vi "M02 Toy Factory.vi"(9 "Angle in":dbl format="%#_13g", 11 "EV3 in":T1) -> (3 "EV3 out":T1)   [LabVIEW 2016]
uses:
  <vilib>/NXT/Subs/LVHSConnector.ctl
  <vilib>/NXT/LegoClasses/BrickReference/BrickReference.lvclass
  <vilib>/NXT/Dual Mode Library/Waits/Wait_Num.vi
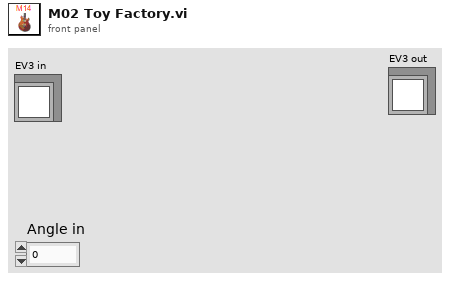
[diagram p1: front panel]
types:
  T1 = typedef "LVHSConnector.ctl" = refnum<class "BrickReference.lvclass">
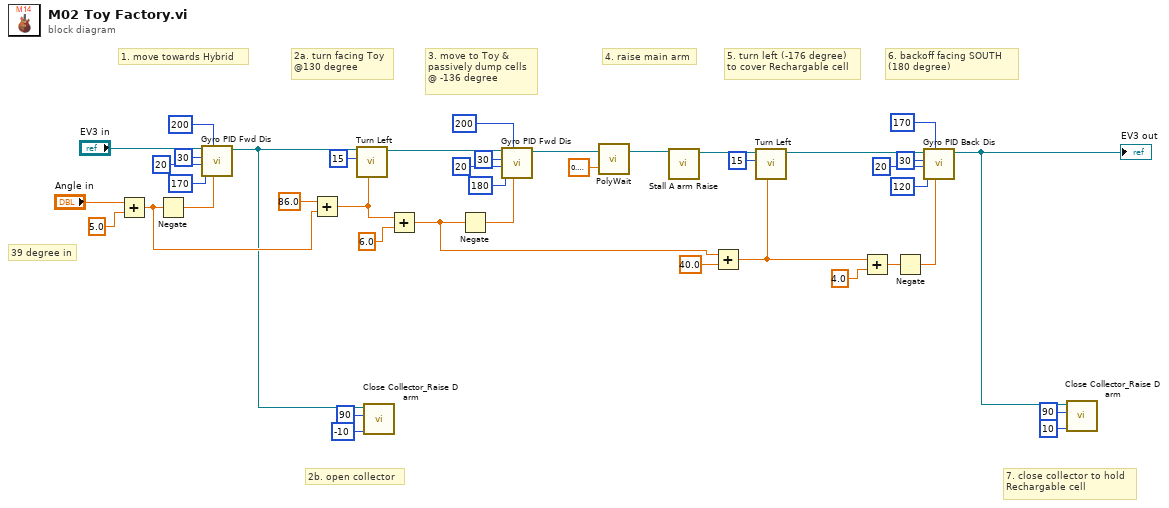
[diagram p0: block diagram]
diagram:
  # "7. close collector to hold\nRechargable cell"
  # "6. backoff facing SOUTH\n(180 degree)"
  # "5. turn left (-176 degree)\nto cover Rechargable cell"
  # "4. raise main arm"
  # "3. move to Toy &\npassively dump cells\n@ -136 degree"
  # "2b. open collector"
  # "2a. turn facing Toy\n@130 degree"
  # "1. move towards Hybrid"
  # "39 degree in"
  n1 = Add(x="Angle in", y=5.0) -> (x+y=w33:dbl)
  n2 = Negate(x=w33) -> (-x=w31:dbl)
  n3 = call "Gyro PID Fwd Dis.vi"("Target angle"=w31, "Threshold to stop"=200 ("Stop rotation"), "Threshold to slow"=170 ("Threshold to De-acc"), "Min. speed"=20 ("De-acc"), "Max. speed"=30 ("Acc"), "EV3 in"="EV3 in") -> ("EV3 out"=w1:T1)  [unwired: 5 in]
  n4 = Add(x=86.0, y=w33) -> (x+y=w39:dbl)
  n5 = call "Turn Left.vi"("Turning angle"=w39, "Motor B (right)"=i8 15, "EV3 in"=w1) -> ("EV3 out"=w26:T1)  [unwired: 8 in]
  n6 = call "Close Collector_Raise D arm.vi"("Power"=i8 -10, "Rotation"=90, "EV3 in"=w1) -> ()  [unwired: 8 in, 1 out]
  n7 = Add(x=w39, y=6.0) -> (x+y=w16:dbl)
  n8 = Negate(x=w16) -> (-x=w18:dbl)
  n9 = call "Gyro PID Fwd Dis.vi"("Target angle"=w18, "Threshold to stop"=200 ("Stop rotation"), "Threshold to slow"=180 ("Threshold to De-acc"), "Min. speed"=20 ("De-acc"), "Max. speed"=30 ("Acc"), "EV3 in"=w26) -> ("EV3 out"=w25:T1)  [unwired: 5 in]
  n10 = call-poly <vilib>:"PolyWait.vi"("Time (1 sec)"=sgl 0.3, "NXT/EV3"=w25) -> ("NXT/EV3"=w21:T1)  [unwired: 2 in]
  n11 = call "Stall A arm Raise.vi"("NXT/EV3"=w21) -> ("NXT/EV3"=w24:T1)  [unwired: 10 in]
  n12 = Add(x=w16, y=40.0) -> (x+y=w9:dbl)
  n13 = call "Turn Left.vi"("Turning angle"=w9, "Motor B (right)"=i8 15, "EV3 in"=w24) -> ("EV3 out"=w15:T1)  [unwired: 8 in]
  n14 = Add(x=w9, y=4.0) -> (x+y=w8:dbl)
  n15 = Negate(x=w8) -> (-x=w7:dbl)
  n16 = call "Gyro PID Back Dis.vi"("Target angle"=w7, "Threshold to stop"=170, "Threshold to slow"=120, "Min. speed"=20, "Max. speed"=30, "EV3 in"=w15) -> ("EV3 out"=w5:T1)  [unwired: 5 in]
  "EV3 out" <- w5
  n17 = call "Close Collector_Raise D arm.vi"("Power"=i8 10, "Rotation"=90, "EV3 in"=w5) -> ()  [unwired: 8 in, 1 out]
